vi "Pure Mock Call Template VI.vi"(8 "error in (no error)":errorcluster, 11 "Mock In":refnum<class "Pure Mock.lvclass">) -> (0 "error out":errorcluster, 3 "Mock Out":refnum<class "Pure Mock.lvclass">)   [LabVIEW 2020]
uses:
  Framework/Pure Mock/Pure Mock.lvclass
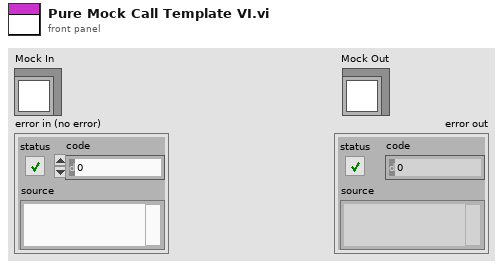
[diagram p1: front panel]
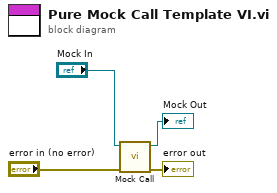
[diagram p0: block diagram]
diagram:
  n1 = call "Mock Call.vi"("error in (no error)"="error in (no error)", "Mock In"="Mock In") -> ("error out"=→"error out":errorcluster, "Mock Out"=→"Mock Out":refnum<class "Pure Mock.lvclass">)  [unwired: 8 in]
